vi "Returning Values By Reference Array Of Simple Struct.vi"(10 "length":i32, 11 "circleArray":cluster{"x":sgl, "y":sgl, "radius":sgl}) -> (3 "circleArray out":cluster{"x":sgl, "y":sgl, "radius":sgl})   [LabVIEW 2018, in "ParsingDataSampleDLL.lvlib"]
doc: "__declspec(dllexport) void ReturningValuesByReference_ArrayOfSimpleStruct (struct simpleStructCircle **circleArray, int length);"
uses:
  ParsingDataSampleDLL.lvlib
  ni_reference_vs/Debug/ParsingDataSampleDLL.dll
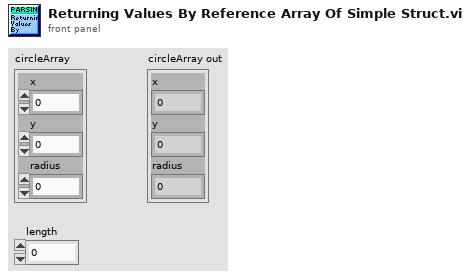
[diagram p1: front panel]
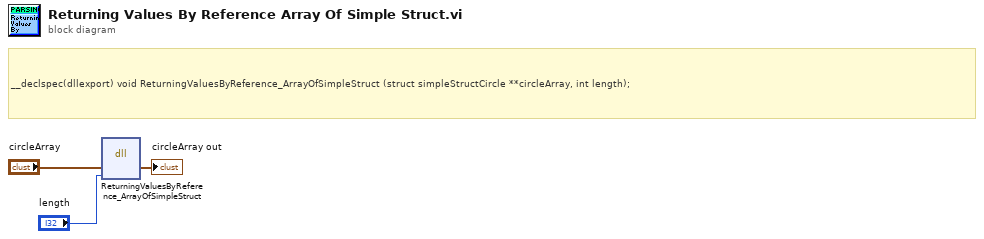
[diagram p0: block diagram]
diagram:
  # "__declspec(dllexport) void ReturningValuesByReference_ArrayOfSimpleStruct (struct simpleStructCircle **circleArray, int length);"
  n1 = dll-call lib="C:/Users/celit/Documents/GitHub/Labview_Python_DLL_Call/ni_reference_vs/Debug/ParsingDataSampleDLL.*" fn="ReturningValuesByReference_ArrayOfSimpleStruct"("circleArray"="circleArray", "length"="length") -> ("circleArray"=→"circleArray out":cluster{"x":sgl, "y":sgl, "radius":sgl})  [unwired: 5 in, 2 out]
